vi "Obtain Thing Shadow.vi"(8 "error in (no error)":errorcluster, 10 "Thing Name":string, 11 "IoT Session in":refnum<class "IoT Session.lvclass">) -> (0 "error out":errorcluster, 2 "Shadow Thing":refnum<class "Thing Shadow.lvclass">, 3 "IoT Session out":refnum<class "IoT Session.lvclass">)   [LabVIEW 2015, in "NI_AWS_IoT.lvlib" / "IoT Session.lvclass"]
uses:
  IoT Session.lvclass
  Thing Shadow/Thing Shadow.lvclass
  Core/HTTP Request/HTTP Request.lvclass/HTTP Request.ctl
  Thing Shadow/Thing Shadow.lvclass/Thing Shadow.ctl
  Core/HTTP Request/Read Credentials.vi
  Core/HTTP Request/Read Verify Server.vi
  Core/HTTP Request/Write Credentials.vi
  Core/HTTP Request/Write Region.vi
  Core/HTTP Request/Write Verify Server.vi
  Core/HTTP Request/Write Service.vi
  Thing Shadow/Write Thing Name.vi
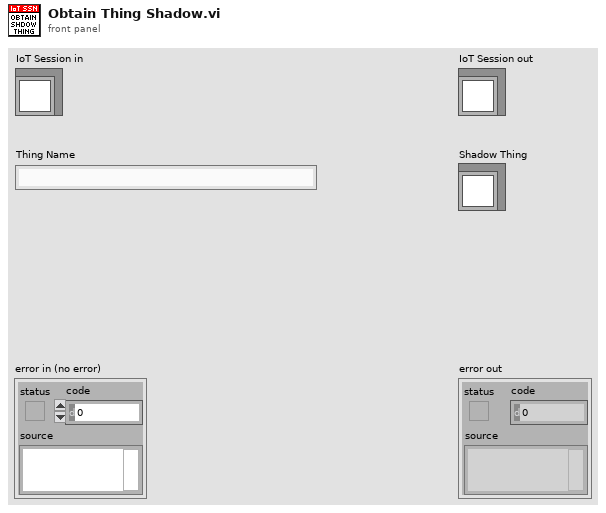
[diagram p1: front panel]
types:
  T1 = typedef "NI_AWS_Core.lvlib/HTTP Request.lvclass/AWS Credentials.ctl" = cluster{"Access Key":string, "Secret Key":string}
  T2 = typedef "NI_AWS_Core.lvlib/HTTP Request.lvclass/Region.ctl" = enum16{"us-east-1", "us-east-2", "us-west-1", "us-west-2", "ap-northeast-1", "ap-northeast-2", "ap-southeast-1", "ap-southeast-2", "ca-central-1", "eu-central-1", "eu-west-1", "eu-west-2", "sa-east-1"}
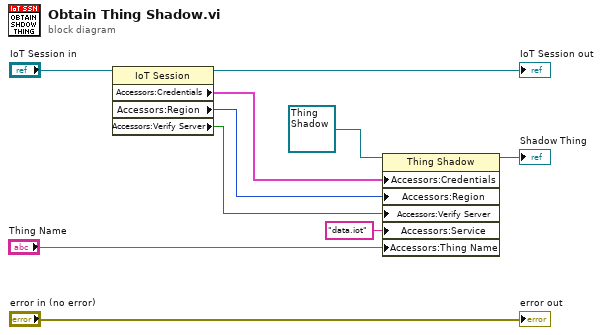
[diagram p0: block diagram]
diagram:
  n1 = property class="IoT Session"(reference="IoT Session in") -> (reference out=→"IoT Session out":refnum<class "IoT Session.lvclass">, "Accessors:Credentials"=w5:T1, "Accessors:Region"=w4:T2, "Accessors:Verify Server"=w3:bool)  [unwired: 1 in, 1 out]
  n2 = property class="Thing Shadow"(reference=refnum<class "Thing Shadow.lvclass"> refnum ("Shadow Thing"), "Accessors:Credentials"=w5, "Accessors:Region"=w4, "Accessors:Verify Server"=w3, "Accessors:Service"="data.iot" ("Service"), "Accessors:Thing Name"="Thing Name") -> (reference out=→"Shadow Thing":refnum<class "Thing Shadow.lvclass">)  [unwired: 1 in, 1 out]
  "error out" <- "error in (no error)"
